vi "Lift_Level_Function.vi"(7 "Level":bool, 8 "upper limit":dbl, 9 "lower Limit":dbl=720.0 format="%#_13g", 10 "MotorControlDevRef":T1={"DeviceStatus"={"status"=FALSE, "code"=0, "source"=""}, "Type"=enum."PWM", "PWM"={"Controller"=enum."Controller 1", "PWM Channel"=enum."Invalid", "DeadBand"={"Name"="", "maxPositivePwm"=0, "minPositivePwm"=0, "centerPwm"=0, "maxNegativePwm"=0, "minNegativePwm"=0, "angularRange"=0}}, "CAN"={"Device Number"=0, "Control Mode"=enum."Percent VBus", "Semaphore"=refnum, "Max Vout"=12.0, "TalonSRX Control Mode"=enum."Percent VBus"}, "Invert"=FALSE, "TransformRef"=refnum, "InvTransformRef"=refnum}, 11 "EncoderDevRef":T10={"DevStatus"={"status"=FALSE, "code"=0, "source"=""}, "EncoderIndex"=enum."Invalid", "CounterIndex"=enum."Invalid", "DistancePerCount"=1.0, "Decoding Type"=enum."4x"}) -> (3 "Level":bool=TRUE)   [LabVIEW 2014]
uses:
  <vilib>/Rock Robotics/SystemInterfaces/Encoder/FPGA_EncoderIdx.ctl
  <vilib>/Rock Robotics/WPI/Encoder/WPI_EncoderType.ctl
  <vilib>/Rock Robotics/SystemInterfaces/Counter/FPGA_CounterCtrSystemIndex.ctl
  <vilib>/Rock Robotics/WPI/Encoder/WPI_EncoderDevRef.ctl
  <vilib>/Rock Robotics/WPI/PWM/WPI_PWMTransform_ConPane.ctl
  <vilib>/Rock Robotics/SystemInterfaces/Typedef/FPGA_TypedefDigitalModule.ctl
  <vilib>/Rock Robotics/SystemInterfaces/DIO/FPGA_DIOPWMChannel.ctl
  <vilib>/Rock Robotics/WPI/PWM/WPI_PWMDeadband.ctl
  <vilib>/Rock Robotics/WPI/CAN/Jaguar/SubVIs/WPI_CANJaguar_ControlMode.ctl
  <vilib>/Rock Robotics/WPI/MotorControl/WPI_MotorControlDeviceRef.ctl
  <vilib>/Rock Robotics/WPI/CAN/TalonSRX/WPI_CANTalonSRX_APIControlMode.ctl
  <vilib>/Rock Robotics/WPI/MotorControl/WPI_MotorControlType.ctl
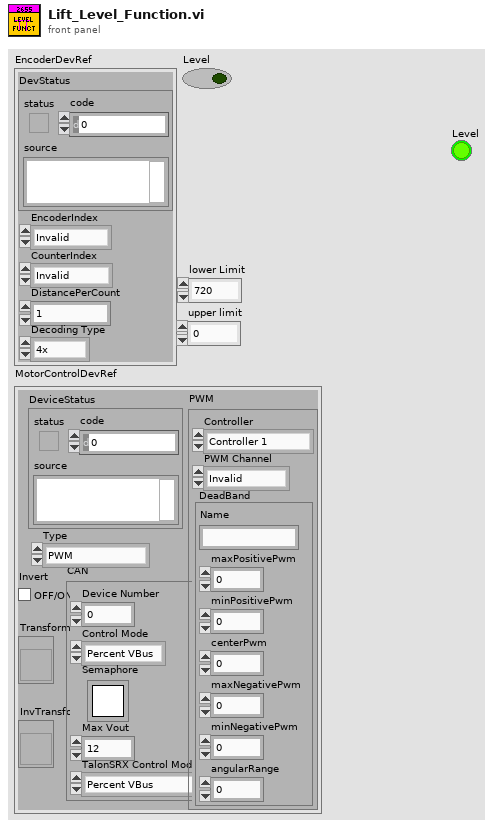
[diagram p1: front panel]
types:
  T1 = typedef "WPI_MotorControlDeviceRef.ctl" = cluster{"DeviceStatus":errorcluster, "Type":T2, "PWM":cluster{"Controller":T3, "PWM Channel":T4, "DeadBand":T5}, "CAN":cluster{"Device Number":u8, "Control Mode":T6, "Semaphore":T7, "Max Vout":dbl, "TalonSRX Control Mode":T8}, "Invert":bool, "TransformRef":T9, "InvTransformRef":T9}
  T2 = typedef "WPI_MotorControlType.ctl" = enum16{"PWM", "CAN", "CANTalonSRX"}
  T3 = typedef "FPGA_TypedefDigitalModule.ctl" = enum16{"Controller 1"}
  T4 = typedef "FPGA_DIOPWMChannel.ctl" = enum8{"PWM 0", "PWM 1", "PWM 2", "PWM 3", "PWM 4", "PWM 5", "PWM 6", "PWM 7", "PWM 8", "PWM 9", "PWM MXP 0", "PWM MXP 1", "PWM MXP 2", "PWM MXP 3", "PWM MXP 4", "PWM MXP 5", "PWM MXP 6", "PWM MXP 7", "PWM MXP 8", "PWM MXP 9", "Invalid"}
  T5 = typedef "WPI_PWMDeadband.ctl" = cluster{"Name":string, "maxPositivePwm":i32, "minPositivePwm":i32, "centerPwm":i32, "maxNegativePwm":i32, "minNegativePwm":i32, "angularRange":u16}
  T6 = typedef "WPI_CANJaguar_ControlMode.ctl" = enum8{"Percent VBus", "Current", "Speed", "Position", "Voltage"}
  T7 = typedef "Semaphore RefNum" = refnum<k1>
  T8 = typedef "WPI_CANTalonSRX_APIControlMode.ctl" = enum8{"Percent VBus", "Speed", "Position", "Slave", "Unchanged / Invalid"}
  T9 = typedef "WPI_PWMTransform_ConPane.ctl" = refnum<vi>
  T10 = typedef "WPI_EncoderDevRef.ctl" = cluster{"DevStatus":errorcluster, "EncoderIndex":T11, "CounterIndex":T12, "DistancePerCount":dbl, "Decoding Type":T13}
  T11 = typedef "FPGA_EncoderIdx.ctl" = enum8{"Enc 0", "Enc 1", "Enc 2", "Enc 3", "Enc 4", "Enc 5", "Enc 6", "Enc 7", "Invalid"}
  T12 = typedef "FPGA_CounterCtrSystemIndex.ctl" = enum8{"Ctr 0", "Ctr 1", "Ctr 2", "Ctr 3", "Ctr 4", "Ctr 5", "Ctr 6", "Ctr 7", "Invalid"}
  T13 = typedef "WPI_EncoderType.ctl" = enum16{"1x", "2x", "4x"}
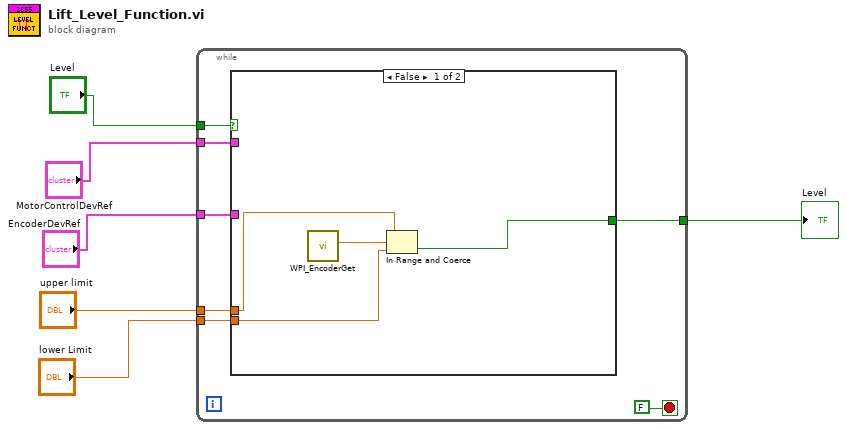
[diagram p0: block diagram]
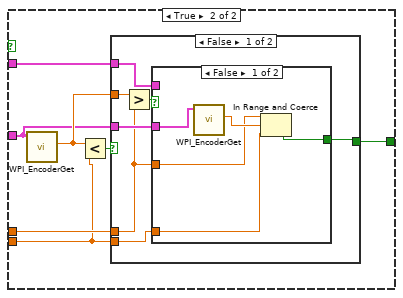
[diagram p2: hidden frame]
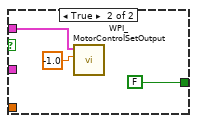
[diagram p3: hidden frame]
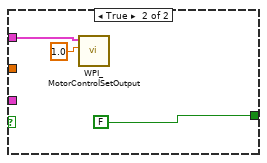
[diagram p4: hidden frame]
diagram:
  n1 = while {
    tunnel: "Level" -> [w12]
    tunnel: "EncoderDevRef" -> [w11]
    tunnel: "MotorControlDevRef" -> [w10]
    tunnel: [w9] -> w3
    tunnel: "lower Limit" -> [w8]
    tunnel: "upper limit" -> [w7]
    stop <- FALSE stop-if-true
    n2 = case shown="False" w12 {
      tunnel: [w17 w23] -> w9
      tunnel: w11 -> [_ w21]
      tunnel: w10 -> [_ w20]
      tunnel: w8 -> [w16 w18]
      tunnel: w7 -> [w14 w19]
      frame False {
        n3 = call <vilib>:"WPI_EncoderGet.vi"() -> ("Distance"=w15:dbl)  [unwired: 6 in, 5 out]
        n4 = In Range and Coerce(upper limit=w14, x=w15, lower limit=w16) -> (In Range?=w17:bool)  [unwired: 1 out]
      }
      frame True {
        n5 = call <vilib>:"WPI_EncoderGet.vi"("EncoderDevRef"=w21) -> ("Distance"=w22:dbl)  [unwired: 5 in, 5 out]
        n6 = Less?(x=w22, y=w18) -> (x < y?=w24:bool)
        n7 = case shown="False" w24 {
          tunnel: [w29 FALSE] -> w23
          tunnel: w22 -> [w31 _]
          tunnel: w21 -> [w28 _]
          tunnel: w20 -> [w27 w40]
          tunnel: w19 -> [w26 _]
          tunnel: w18 -> [w25 _]
          frame False {
            n8 = Greater?(x=w31, y=w26) -> (0:w30:bool)
            n9 = case shown="False" w30 {
              tunnel: [w35 FALSE] -> w29
              tunnel: w28 -> [w36 _]
              tunnel: w27 -> [_ w37]
              tunnel: w26 -> [w32 _]
              tunnel: w25 -> [w33 _]
              frame False {
                n10 = call <vilib>:"WPI_EncoderGet.vi"("EncoderDevRef"=w36) -> ("Distance"=w34:dbl)  [unwired: 5 in, 5 out]
                n11 = In Range and Coerce(upper limit=w32, x=w34, lower limit=w33) -> (In Range?=w35:bool)  [unwired: 1 out]
              }
              frame True {
                n12 = call <vilib>:"WPI_MotorControlSetOutput.vi"("Output"=-1.0, "MotorControlDevRef"=w37) -> ()  [unwired: 7 in, 3 out]
              }
            }
          }
          frame True {
            n13 = call <vilib>:"WPI_MotorControlSetOutput.vi"("Output"=1.0, "MotorControlDevRef"=w40) -> ()  [unwired: 7 in, 3 out]
          }
        }
      }
    }
  }
  "Level" <- w3
